vi "ToolBarButtonDraw_4_AutoFit.vi"(6 "Color":u32(colorbox), 8 "Focus":bool, 9 "Continuous":bool, 10 "rect":T1, 11 "Pict IN":picture) -> (3 "Pict OUT":picture)   [LabVIEW 2020, in "Sgraph_lib_V1.lvlib" / "Gviewer.lvclass"]
doc: "Draw Autoscale Fit icon in button bar"
uses:
  Gviewer.lvclass
  <vilib>/picture/picture.llb/imagedata.ctl
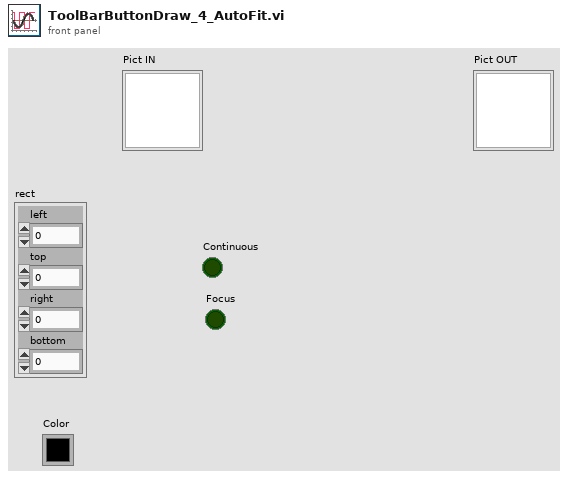
[diagram p1: front panel]
types:
  T1 = cluster{"left":i16, "top":i16, "right":i16, "bottom":i16}
  T2 = typedef "imagedata.ctl" = cluster{"image type":i32, "image depth":i32, "image":u8[], "mask":u8[], "colors":u32[], "Rectangle":cluster{"left":i16, "top":i16, "right":i16, "bottom":i16}}
  T3 = cluster{"horizontal":enum16{"left", "center", "right"}, "vertical":enum16{"top", "center", "bottom"}}
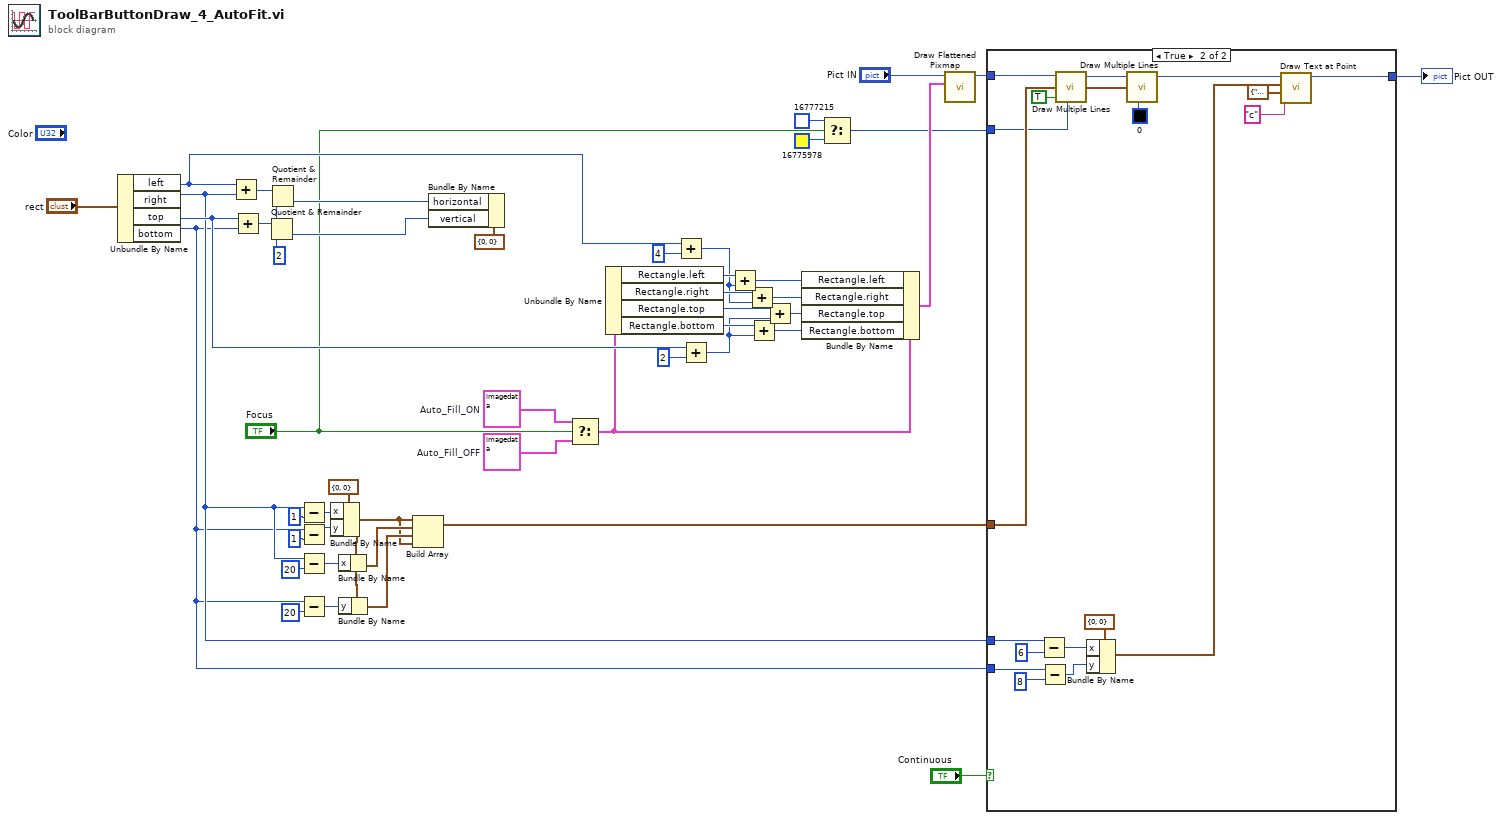
[diagram p0: block diagram]
diagram:
  w18 = T2 {"image type"=0, "image depth"=32, "image"=array[3108 elements], "mask"=[0, 0, 0, 0, 0, 0, 33, 240, 255, 195, 224, 0, 113, 240, 255, 195, 224, 0, 248, 120, 129, 226, 0, 0, 32, 204, 129, 50, 0, 0, 32, 204, 129, 50, 0, 0, 32, 204, 131, 50, 0, 0, 33, 198, 135, 26, 0, 0, 33, 198, 135, 26, 0, 0, 33, 198, 135, 26, 0, 0, 32, 67, 141, 14, 0, 0, 32, 67, 141, 14, 0, 0, 32, 67, 141, 14, 0, 0, 32, 67, 141, 14, 0, 0, 32, 65, 153, 6, 96, 0, 32, 65, 153, 6, 96, 0, 32, 65, 153, 6, 96, 0, 248, 64, 241, 3, 192, 0, 112, 127, 225, 255, 128, 0, 32, 127, 225, 255, 128, 0, 0, 0, 0, 0, 0, 0], "colors"=[], "Rectangle"={"left"=0, "top"=0, "right"=37, "bottom"=21}}  # Auto_Fill_ON
  w19 = T2 {"image type"=0, "image depth"=32, "image"=array[3108 elements], "mask"=[0, 0, 0, 0, 0, 0, 33, 240, 255, 195, 224, 0, 113, 240, 255, 195, 224, 0, 248, 120, 129, 226, 0, 0, 32, 204, 129, 50, 0, 0, 32, 204, 129, 50, 0, 0, 32, 204, 131, 50, 0, 0, 33, 198, 135, 26, 0, 0, 33, 198, 135, 26, 0, 0, 33, 198, 135, 26, 0, 0, 32, 67, 141, 14, 0, 0, 32, 67, 141, 14, 0, 0, 32, 67, 141, 14, 0, 0, 32, 67, 141, 14, 0, 0, 32, 65, 153, 6, 96, 0, 32, 65, 153, 6, 96, 0, 32, 65, 153, 6, 96, 0, 248, 64, 241, 3, 192, 0, 112, 127, 225, 255, 128, 0, 32, 127, 225, 255, 128, 0, 0, 0, 0, 0, 0, 0], "colors"=[], "Rectangle"={"left"=0, "top"=0, "right"=37, "bottom"=21}}  # Auto_Fill_OFF
  w45 = i16 2 ("y")
  n1 = Unbundle By Name("rect") -> ("left"=w29:i16, "right"=w2:i16, "top"=w20:i16, "bottom"=w1:i16)
  n2 = Add(x=w29, y=w2) -> (x+y=w47:i16)
  n3 = Add(x=w20, y=w1) -> (x+y=w46:i16)
  n4 = Quotient & Remainder(x=w46, y=w45) -> (floor(x/y)=w38:i16)  [unwired: 1 out]
  n5 = Quotient & Remainder(x=w47, y=w45) -> (floor(x/y)=w37:i16)  [unwired: 1 out]
  n6 = Subtract(x=w2, y=i16 1) -> (x-y=w42:i16)
  n7 = Subtract(x=w1, y=i16 1) -> (x-y=w12:i16)
  n8 = Subtract(x=w2, y=i16 20) -> (x-y=w40:i16)
  n9 = Subtract(x=w1, y=i16 20) -> (x-y=w11:i16)
  n10 = Bundle By Name(cluster=cluster{"x":i16, "y":i16} {"x"=0, "y"=0}, "x"=w42, "y"=w12) -> (w8:cluster{"x":i16, "y":i16})
  n11 = Bundle By Name(cluster=w8, "x"=w40) -> (w39:cluster{"x":i16, "y":i16})
  n12 = Bundle By Name(cluster=w8, "y"=w11) -> (w9:cluster{"x":i16, "y":i16})
  n13 = Build Array(w8, w39, w9, w8) -> (w15:cluster{"x":i16, "y":i16}[])
  n14 = Bundle By Name(cluster=cluster{"horizontal":i16, "vertical":i16} {"horizontal"=0, "vertical"=0} ("pixel center"), "horizontal"=w37, "vertical"=w38) -> ()  [unwired: 1 out]
  n15 = Select(t=w18, s="Focus", f=w19) -> (s? t:f=w17:T2)
  n16 = Unbundle By Name(w17) -> ("Rectangle.left"=w33:i16, "Rectangle.right"=w32:i16, "Rectangle.top"=w31:i16, "Rectangle.bottom"=w30:i16)
  n17 = Add(x=w29, y=i16 4) -> (x+y=w28:i16)
  n18 = Add(x=w20, y=i16 2) -> (x+y=w25:i16)
  n19 = Add(x=w33, y=w28) -> (x+y=w21:i16)
  n20 = Add(x=w32, y=w28) -> (x+y=w22:i16)
  n21 = Add(x=w30, y=w25) -> (x+y=w23:i16)
  n22 = Add(x=w31, y=w25) -> (x+y=w24:i16)
  n23 = Bundle By Name(cluster=w17, "Rectangle.left"=w21, "Rectangle.right"=w22, "Rectangle.top"=w24, "Rectangle.bottom"=w23) -> (w34:T2)
  n24 = Select(t=u32 16777215 ("color(black)"), s="Focus", f=u32 16775978 ("color(black)")) -> (s? t:f=w4:u32)
  n25 = call <vilib>:"Draw Flattened Pixmap.vi"("image data"=w34, "picture"="Pict IN") -> ("new picture"=w16:picture)  [unwired: 7 in]
  n26 = case shown="True" "Continuous" {
    tunnel: w16 -> [w49 w67]
    tunnel: w15 -> [_ w65]
    tunnel: [w49 w54] -> w14
    tunnel: w4 -> [_ w62]
    tunnel: w2 -> [_ w60]
    tunnel: w1 -> [_ w59]
    frame False {
    }
    frame True {
      n27 = Subtract(x=w60, y=i16 6) -> (x-y=w57:i16)
      n28 = Subtract(x=w59, y=i16 8) -> (x-y=w56:i16)
      n29 = call <vilib>:"Draw Multiple Lines.vi"("picture"=w67, "line endpoints"=w65, "fill?(F)"=TRUE, "color(black)"=w62) -> ("new picture"=w64:picture)  [unwired: 5 in]
      n30 = Bundle By Name(cluster=cluster{"x":i16, "y":i16} {"x"=0, "y"=0}, "x"=w57, "y"=w56) -> (w53:cluster{"x":i16, "y":i16})
      n31 = call <vilib>:"Draw Multiple Lines.vi"("picture"=w64, "line endpoints"=w65, "color(black)"=u32 0) -> ("new picture"=w55:picture)  [unwired: 6 in]
      n32 = call <vilib>:"Draw Text at Point.vi"("text"="c", "alignment(left, top)"=T3 {"horizontal"=enum."center", "vertical"=enum."center"}, "origin"=w53, "picture"=w55) -> ("new picture"=w54:picture)  [unwired: 6 in, 1 out]
    }
  }
  "Pict OUT" <- w14
